vi "read_P_liq0.vi"() -> (3 "Actual P liq Flow Rate":dbl, 4 "P liq Remote":bool, 5 "P liq Run":bool, 6 "P liq Bubbler":bool, 7 "P liq Active":bool)   [LabVIEW 2011]
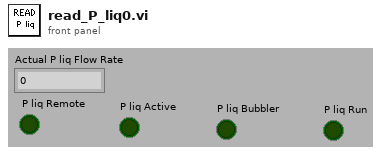
[diagram p1: front panel]
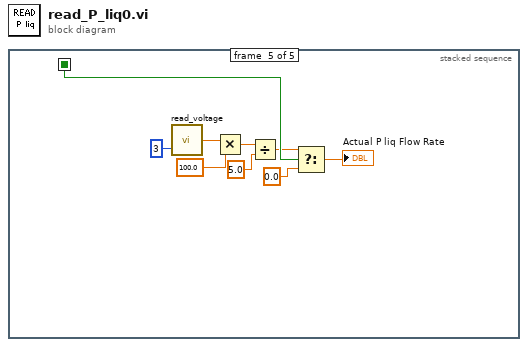
[diagram p0: block diagram]
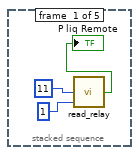
[diagram p2: hidden frame]
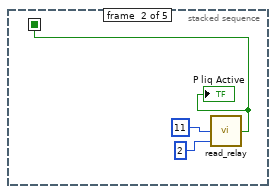
[diagram p3: hidden frame]
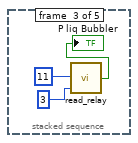
[diagram p4: hidden frame]
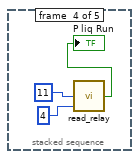
[diagram p5: hidden frame]
diagram:
  n1 = stacked-sequence {
    seq-local: [_ w4 _ _ _] -> [_ _ _ _ w16]
    frame #0 {
      n2 = call "read_relay.vi"("Relay"=1, "Slot"=11) -> ("Relay Status"=→"P liq Remote":bool)  [unwired: 1 out]
    }
    frame #1 {
      n3 = call "read_relay.vi"("Relay"=2, "Slot"=11) -> ("Relay Status"=w4:bool)  [unwired: 1 out]
      "P liq Active" <- w4
    }
    frame #2 {
      n4 = call "read_relay.vi"("Relay"=3, "Slot"=11) -> ("Relay Status"=→"P liq Bubbler":bool)  [unwired: 1 out]
    }
    frame #3 {
      n5 = call "read_relay.vi"("Relay"=4, "Slot"=11) -> ("Relay Status"=→"P liq Run":bool)  [unwired: 1 out]
    }
    frame #4 {
      n6 = call "read_voltage.vi"("Channel"=3) -> ("Voltage"=w20:dbl)  [unwired: 1 in]
      n7 = Multiply(x=w20, y=100.0) -> (x*y=w18:dbl)
      n8 = Divide(x=w18, y=5.0) -> (x/y=w15:dbl)
      n9 = Select(t=w15, s=w16, f=0.0) -> (s? t:f=→"Actual P liq Flow Rate":dbl)
    }
  }
